vi "Create Normal.vi"(7 "3D Surface Property":T1={"General Property"={"Plot Name"="", "Coordinate System"=enum."Cartesian", "Opacity"=0.0}, "Projection Property"={"Draw XY"=FALSE, "Draw YZ"=FALSE, "Draw XZ"=FALSE}, "Plot Property"={"Draw Surface"=FALSE, "Draw Mesh"=FALSE, "Draw Normal"=FALSE, "Color Ramp Cluster"={"Color Ramp Style"=enum."None", "Color Ramp Array"=[16711934, 393471, 57855, 4390754, 16449346, 16744722, 16711680], "Color Ramp Index"=[45, 91, 133, 175, 219, 255], "Interpolate?"=FALSE, "Logarithm?"=FALSE}, "Line Style"=enum."None", "Line Width"=0.0, "Line Color"=0, "Antialiasing"=FALSE}, "Surface Property"={"Color Mode"=enum."Flat Shading"}}, 8 "error in (no error)":errorcluster, 9 "Actual Transform In":T4, 10 "Plot Representation In":T6, 11 "Plot Object In":refnum<vi>) -> (0 "error out":errorcluster, 1 "Actual Transform Out":T4, 2 "Plot Representation Out":T6, 3 "Plot Object Out":refnum<vi>, 4 "Normal Object Out":refnum<vi>)   [LabVIEW 2020, in "3D Surface.lvclass"]
uses:
  3D Surface.lvclass
  Plot Representation.ctl
  Range Clusters.ctl
  Mesh Data.ctl
  Actual Transform.ctl
  3D Surface Property.ctl
  Color Ramp Cluster.ctl
  Line Type.ctl
  3D Plot.lvclass
  NI_3D Picture Control.lvlib
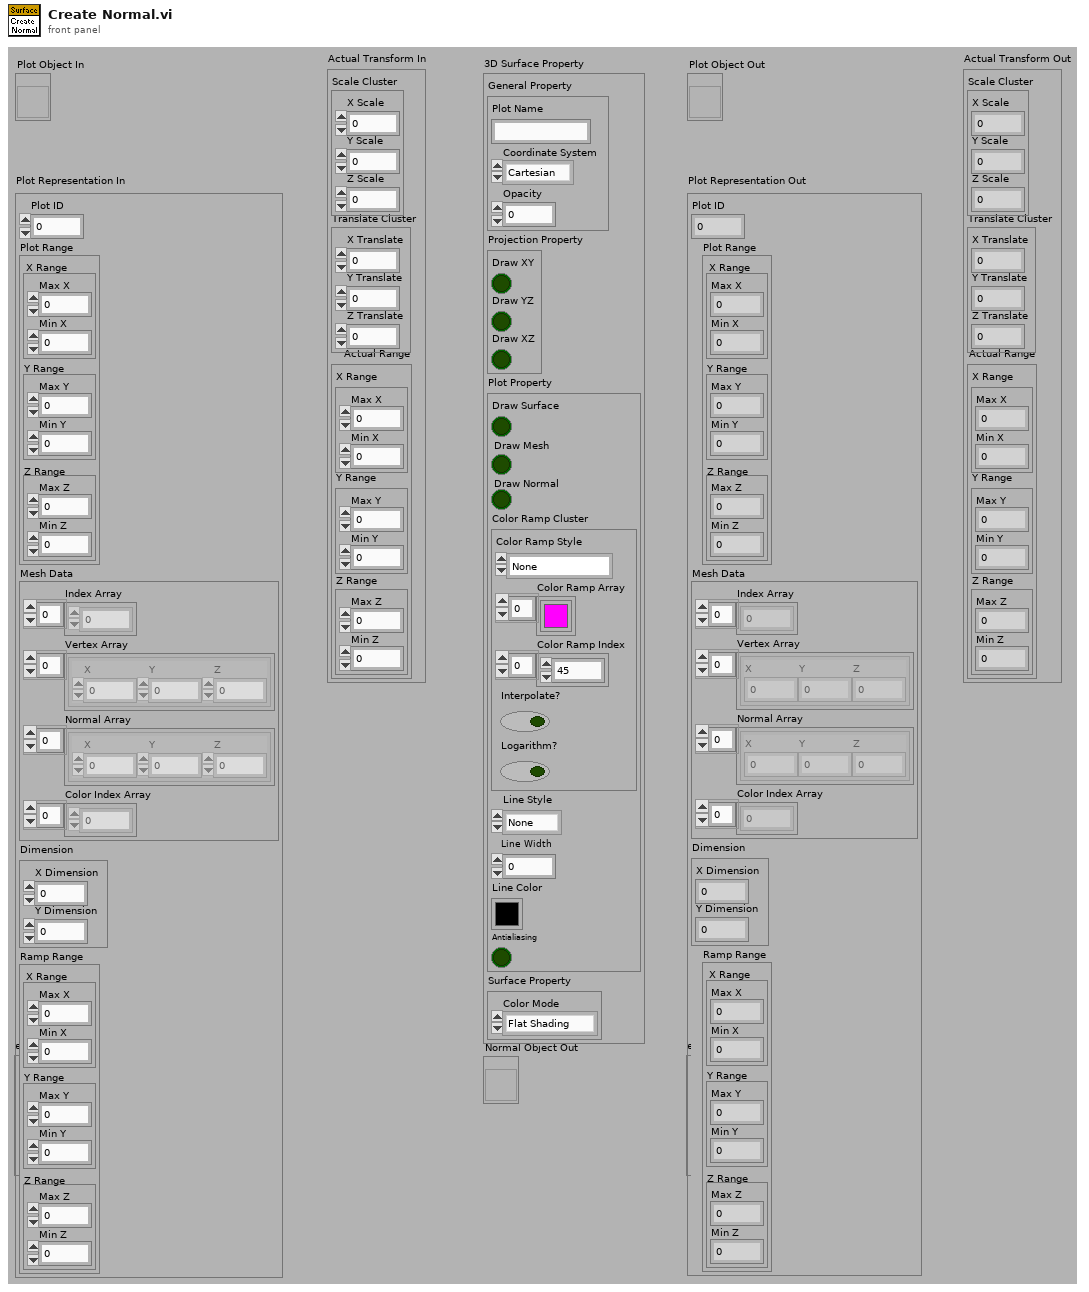
[diagram p1: front panel]
types:
  T1 = typedef "3D Surface.lvclass/3D Surface Property.ctl" = cluster{"General Property":cluster{"Plot Name":string, "Coordinate System":enum16{"Cartesian", "Cylindrical", "Spherical"}, "Opacity":sgl}, "Projection Property":cluster{"Draw XY":bool, "Draw YZ":bool, "Draw XZ":bool}, "Plot Property":cluster{"Draw Surface":bool, "Draw Mesh":bool, "Draw Normal":bool, "Color Ramp Cluster":T2, "Line Style":T3, "Line Width":sgl, "Line Color":u32, "Antialiasing":bool}, "Surface Property":cluster{"Color Mode":enum16{"Flat Shading", "Interpolated Shading"}}}
  T2 = typedef "3D Plot.lvclass/Color Ramp Cluster.ctl" = cluster{"Color Ramp Style":enum16{"None", "Shaded", "Color spectrum", "Grey scale", "Custom"}, "Color Ramp Array":u32[], "Color Ramp Index":i32[], "Interpolate?":bool, "Logarithm?":bool}
  T3 = typedef "3D Plot.lvclass/Line Type.ctl" = enum16{"None", "Solid", "Dash", "Dot", "Dash Dot"}
  T4 = typedef "3D Plot.lvclass/Actual Transform.ctl" = cluster{"Scale Cluster":cluster{"X Scale":sgl, "Y Scale":sgl, "Z Scale":sgl}, "Translate Cluster":cluster{"X Translate":sgl, "Y Translate":sgl, "Z Translate":sgl}, "Actual Range":T5}
  T5 = typedef "3D Plot.lvclass/Range Clusters.ctl" = cluster{"X Range":cluster{"Max X":sgl, "Min X":sgl}, "Y Range":cluster{"Max Y":sgl, "Min Y":sgl}, "Z Range":cluster{"Max Z":sgl, "Min Z":sgl}}
  T6 = typedef "3D Plot.lvclass/Plot Representation.ctl" = cluster{"Plot ID":i32, "Plot Range":T5, "Mesh Data":T7, "Dimension":cluster{"X Dimension":i32, "Y Dimension":i32}, "Ramp Range":T5}
  T7 = typedef "3D Plot.lvclass/Mesh Data.ctl" = cluster{"Index Array":u32[], "Vertex Array":cluster{"X":sgl, "Y":sgl, "Z":sgl}[], "Normal Array":cluster{"X":sgl, "Y":sgl, "Z":sgl}[], "Color Index Array":i32[]}
  T8 = enum16{"Overall", "Per Primitive", "Per Vertex", "Binding Off"}
  T9 = enum16{"Points", "Lines", "Line Strip", "Line Loop", "Triangles", "Triangle Strip", "Triangle Fan", "Quads", "Quad Strip", "Polygon"}
  T10 = cluster{"X Scale":sgl, "Y Scale":sgl, "Z Scale":sgl}
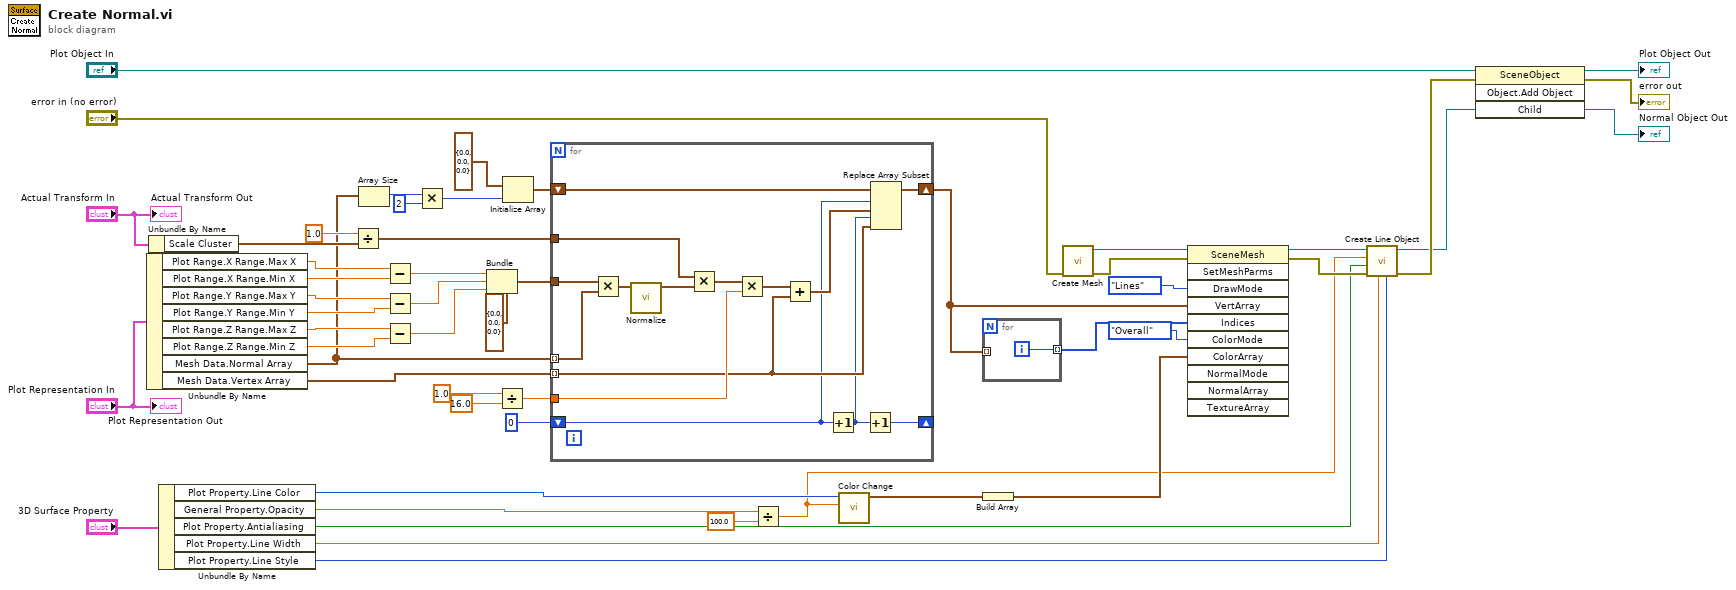
[diagram p0: block diagram]
diagram:
  n1 = Unbundle By Name("Plot Representation In") -> ("Plot Range.X Range.Max X"=w27:sgl, "Plot Range.X Range.Min X"=w26:sgl, "Plot Range.Y Range.Max Y"=w25:sgl, "Plot Range.Y Range.Min Y"=w24:sgl, "Plot Range.Z Range.Max Z"=w23:sgl, "Plot Range.Z Range.Min Z"=w22:sgl, "Mesh Data.Normal Array"=w9:cluster{"X":sgl, "Y":sgl, "Z":sgl}[], "Mesh Data.Vertex Array"=w14:cluster{"X":sgl, "Y":sgl, "Z":sgl}[])
  n2 = Unbundle By Name("Actual Transform In") -> ("Scale Cluster"=w34:T10)
  n3 = Unbundle By Name("3D Surface Property") -> ("Plot Property.Line Color"=w31:u32, "General Property.Opacity"=w17:sgl, "Plot Property.Antialiasing"=w20:bool, "Plot Property.Line Width"=w19:sgl, "Plot Property.Line Style"=w21:T3)
  n4 = Divide(x=sgl 1.0, y=w34) -> (x/y=w32:T10)
  n5 = Array Size(array=w9) -> (size(s)=w8:i32)
  n6 = Subtract(x=w27, y=w26) -> (x-y=w36:sgl)
  n7 = Subtract(x=w25, y=w24) -> (x-y=w37:sgl)
  n8 = Subtract(x=w23, y=w22) -> (x-y=w38:sgl)
  n9 = Multiply(x=w8, y=2) -> (x*y=w7:i32)
  n10 = Bundle(cluster=cluster{"X":sgl, "Y":sgl, "Z":sgl} {"X"=0.0, "Y"=0.0, "Z"=0.0} ("Vector"), "X"=w36, "Y"=w37, "Z"=w38) -> (w52:cluster{"X":sgl, "Y":sgl, "Z":sgl})
  n11 = Divide(x=sgl 1.0, y=sgl 16.0) -> (x/y=w35:sgl)
  n12 = Initialize Array(cluster{"X":sgl, "Y":sgl, "Z":sgl} {"X"=0.0, "Y"=0.0, "Z"=0.0} ("3D Point"), w7) -> (w11:cluster{"X":sgl, "Y":sgl, "Z":sgl}[])
  n13 = for {
    tunnel: w9 -> [w66] mode=indexing
    tunnel: w14 -> [w56] mode=indexing
    tunnel: w52 -> [w67]
    tunnel: w35 -> [w64]
    shift-right: [w58] -> w12
    shift-left: w11 -> [w59]
    tunnel: w32 -> [w60]
    shift-right: [w55] -> _
    shift-left: 0 ("y") -> [w53]
    n14 = Multiply(x=w67, y=w66) -> (x*y=w65:cluster{"X":sgl, "Y":sgl, "Z":sgl})
    n15 = call "Normalize.vi"("Vector"=w65) -> ("Normalized Vector"=w62:cluster{"X":sgl, "Y":sgl, "Z":sgl})  [unwired: 10 out]
    n16 = Multiply(x=w60, y=w62) -> (x*y=w61:cluster{sgl, sgl, sgl})
    n17 = Multiply(x=w61, y=w64) -> (x*y=w63:cluster{sgl, sgl, sgl})
    n18 = Add(x=w63, y=w56) -> (x+y=w57:cluster{sgl, sgl, sgl})
    n19 = Increment(x=w53) -> (x+1=w54:i32)
    n20 = Increment(x=w54) -> (x+1=w55:i32)
    n21 = Replace Array Subset(array=w59, new element #1=w57, index #1=w53, new element #2=w56, index #2=w54) -> (w58:cluster{"X":sgl, "Y":sgl, "Z":sgl}[])
  }
  n22 = Divide(x=w17, y=sgl 100.0) -> (x/y=w16:sgl)
  n23 = call "Color Change.vi"("Alpha"=w16, "Color"=w31) -> ("RGBA"=w48:cluster{"R":sgl, "G":sgl, "B":sgl, "A":sgl})  [unwired: 9 out]
  n24 = for {
    tunnel: [w68] -> w13 mode=indexing
    tunnel: w12 -> [_] mode=indexing
    i -> [w68]
  }
  n25 = Build Array(w48) -> (w28:cluster{"R":sgl, "G":sgl, "B":sgl, "A":sgl}[])
  n26 = call "Create Mesh.vi"("error in (no error)"="error in (no error)") -> ("error out"=w47:errorcluster, "New Mesh Refnum"=w50:refnum<vi>)  [unwired: 9 out]
  n27 = invoke class="SceneMesh" method="SetMeshParms"(reference=w50, error in=w47, "DrawMode"=T9."Lines" ("Draw Mode"), "VertArray"=w12, "Indices"=w13, "ColorMode"=T8."Overall" ("Color Binding Mode"), "ColorArray"=w28) -> (reference out=w30:refnum<vi>, error out=w29:errorcluster)  [unwired: 4 in, 9 out]
  n28 = call "Create Line Object.vi"("Line Style"=w21, "Line Width"=w19, "error in (no error)"=w29, "Antialiasing"=w20, "Alpha"=w16, "Mesh Ref In"=w30) -> ("error out"=w4:errorcluster, "Object Ref Out"=w3:refnum<vi>)  [unwired: 4 out]
  n29 = invoke class="SceneObject" method="Object.Add Object"(reference="Plot Object In", error in=w4, "Child"=w3) -> (reference out=→"Plot Object Out":refnum<vi>, error out=→"error out":errorcluster, "Child"=→"Normal Object Out":refnum<vi>)  [unwired: 1 in, 1 out]
  "Plot Representation Out" <- "Plot Representation In"
  "Actual Transform Out" <- "Actual Transform In"
